vi "_Parse SEM Result.vi"(8 "error in (no error)":errorcluster, 10 "Input String":string, 11 "VISA resource name":refnum<visa-resource-name>) -> (0 "error out":errorcluster, 1 "Measurement Result":T1 {"TX Power" format="%^.3e"; "OBW" format="%^.3e"; "Out Of Tolerance" format="%^.3e"}, 2 "Reliability":i32, 3 "VISA resource name out":refnum<visa-resource-name>)   [LabVIEW 2015, in "Rohde&Schwarz CMXP NR FR2 Measurement.lvlib"]
uses:
  <instrlib>/Rohde&Schwarz CMXP NR FR2 Measurement/Rohde&Schwarz CMXP NR FR2 Measurement.lvlib
  <instrlib>/Rohde&Schwarz CMXP NR FR2 Measurement/Private/rsidr_core.llb/rsidr_core.lvlib
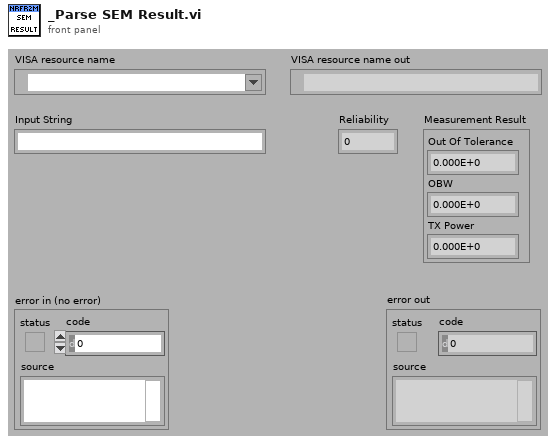
[diagram p1: front panel]
types:
  T1 = cluster{"Out Of Tolerance":dbl, "OBW":dbl, "TX Power":dbl}
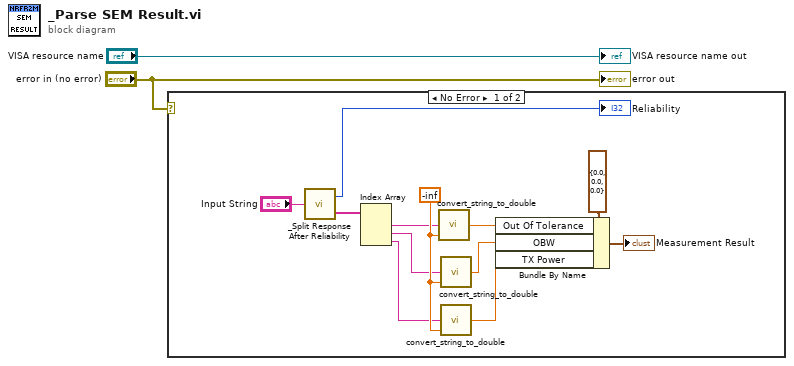
[diagram p0: block diagram]
diagram:
  n1 = case shown="No Error" "error in (no error)" {
    frame No Error {
      w14 = -inf
      n2 = call <instrlib>:"_Split Response After Reliability.vi"("Input String"="Input String") -> ("Response out"=w7:string[], "Reliability out"=→"Reliability":i32)
      n3 = Index Array(array=w7) -> (element #1=w6:string, element #2=w5:string, element #3=w4:string)  [unwired: 3 in]
      n4 = call <instrlib>:"convert_string_to_double.vi"("default (0)"=w14, "String in"=w6) -> ("double value out"=w12:dbl)  [unwired: 3 in]
      n5 = call <instrlib>:"convert_string_to_double.vi"("default (0)"=w14, "String in"=w5) -> ("double value out"=w11:dbl)  [unwired: 3 in]
      n6 = call <instrlib>:"convert_string_to_double.vi"("default (0)"=w14, "String in"=w4) -> ("double value out"=w10:dbl)  [unwired: 3 in]
      n7 = Bundle By Name(cluster=T1 {"Out Of Tolerance"=0.0, "OBW"=0.0, "TX Power"=0.0} ("Measurement Result"), "Out Of Tolerance"=w12, "OBW"=w11, "TX Power"=w10) -> (→"Measurement Result":T1)
    }
    frame Error {
    }
  }
  "error out" <- "error in (no error)"
  "VISA resource name out" <- "VISA resource name"
